vi "New Picture Update.vi"(11 "Frame Reference":refnum<vi>) -> (3 "Updated Picture":picture)   [LabVIEW 2020]
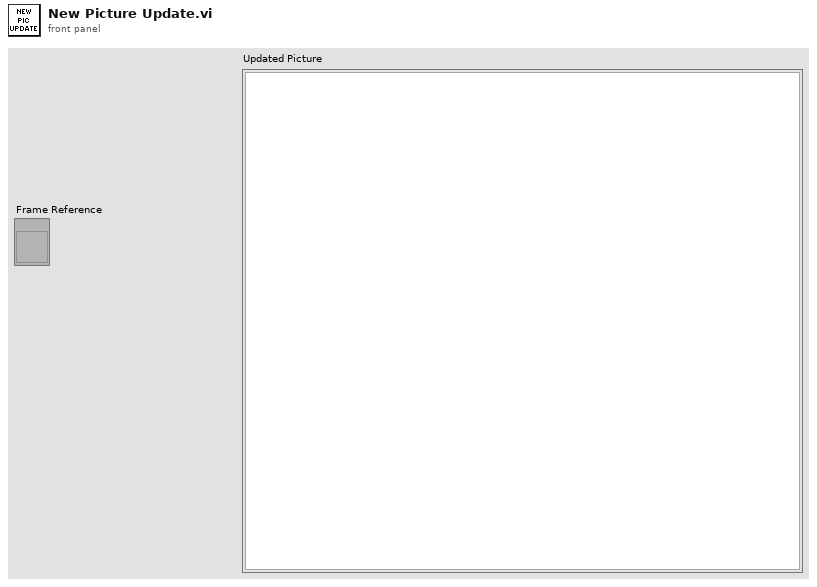
[diagram p1: front panel]
types:
  T1 = typedef "LVBoundsTypeDef.ctl" = cluster{"Width":u32, "Height":u32}
  T2 = typedef "imagedata.ctl" = cluster{"image type":i32, "image depth":i32, "image":u8[], "mask":u8[], "colors":u32[], "Rectangle":cluster{"left":i16, "top":i16, "right":i16, "bottom":i16}}
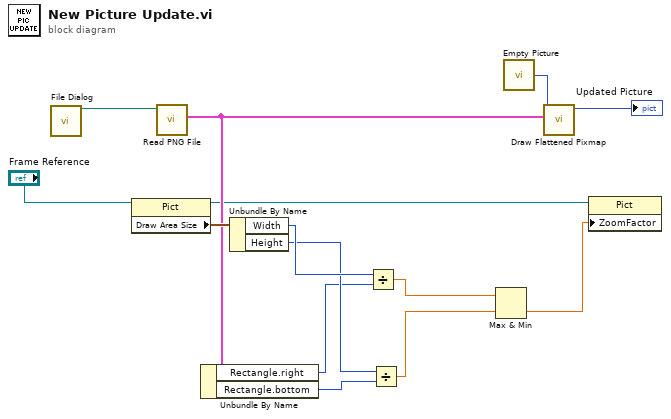
[diagram p0: block diagram]
diagram:
  n1 = call "File Dialog"() -> ("selected path"=w14:path)  [unwired: 12 in, 3 out]
  n2 = property class="Pict"(reference="Frame Reference") -> (reference out=w1:refnum<vi>, "Draw Area Size"=w10:T1)  [unwired: 1 in, 1 out]
  n3 = call <vilib>:"Read PNG File.vi"("path to PNG file"=w14) -> ("image data"=w5:T2)  [unwired: 8 in, 2 out]
  n4 = Unbundle By Name(w5) -> ("Rectangle.right"=w6:i16, "Rectangle.bottom"=w7:i16)
  n5 = Unbundle By Name(w10) -> ("Width"=w9:u32, "Height"=w8:u32)
  n6 = Divide(x=w9, y=w6) -> (x/y=w4:dbl)
  n7 = Divide(x=w8, y=w7) -> (x/y=w3:dbl)
  n8 = Max & Min(x=w4, y=w3) -> (min(x,y)=w2:dbl)  [unwired: 1 out]
  n9 = call "Empty Picture"() -> ("empty picture"=w13:picture)
  n10 = call <vilib>:"Draw Flattened Pixmap.vi"("image data"=w5, "picture"=w13) -> ("new picture"=→"Updated Picture":picture)  [unwired: 7 in]
  n11 = property class="Pict"(reference=w1, "ZoomFactor"=w2) -> ()  [unwired: 1 in, 2 out]
